vi "GetLocalClassPath.vi"(1 "full class name":string, 5 "error in (no error)":errorcluster) -> (15 "local class path":path, 16 "found?":bool, 19 "error out":errorcluster)   [LabVIEW 2017, in "G#RemoteProxy.lvclass"]
doc: "Returns the local class path on the computer."
uses:
  G#RemoteProxy.lvclass
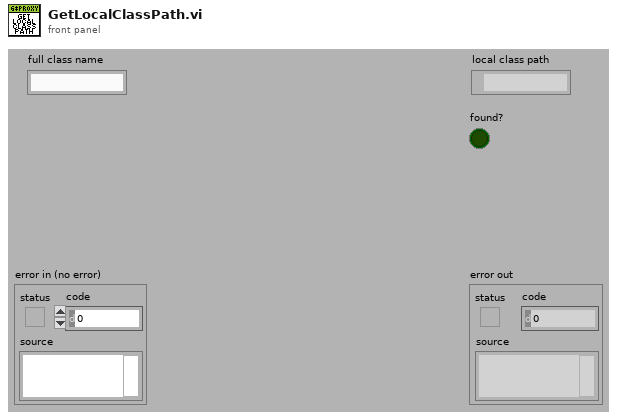
[diagram p1: front panel]
types:
  T1 = typedef "G#RemoteProxy.lvclass/ClassAttributesProxy.ctl" = cluster{"NoActiveProject":bool, "FullClassNames":string[], "FullClassPaths":path[], "RemoteRefs":refnum<class "G#Object.lvclass">[], "ProxyRefs":refnum<class "G#RemoteProxy.lvclass">[], "RemoteClassName":string[], "ProxyClassRefs":refnum<class "G#RemoteProxy.lvclass">[]}
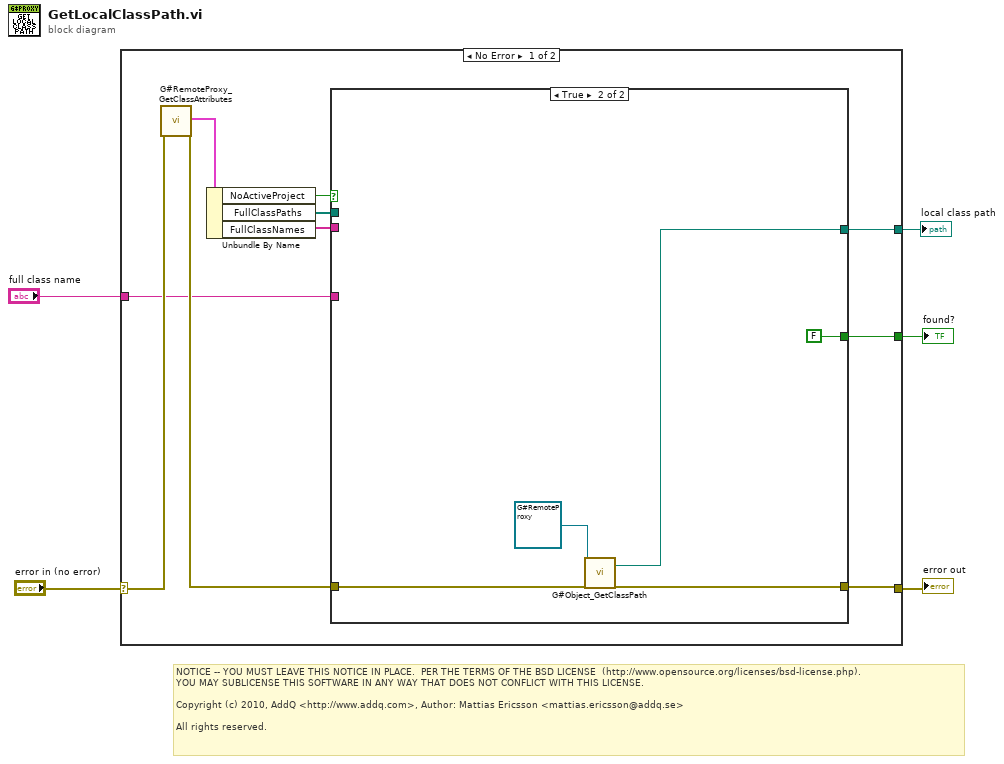
[diagram p0: block diagram]
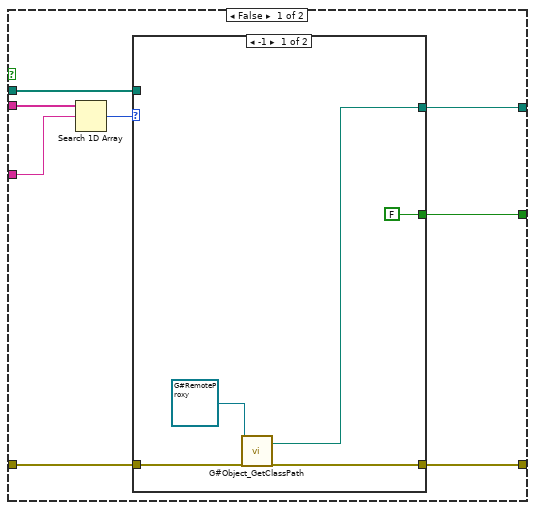
[diagram p2: hidden frame]
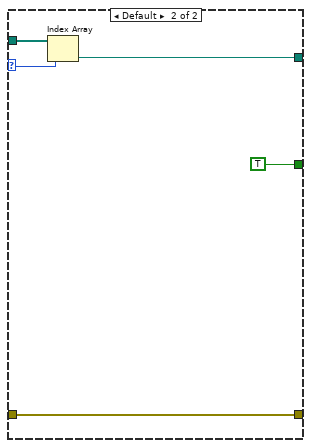
[diagram p3: hidden frame]
diagram:
  # "NOTICE -- YOU MUST LEAVE THIS NOTICE IN PLACE.  PER THE TERMS OF THE BSD LICENSE  (http://www.opensource.org/licenses/bsd-license.php).\nYOU MAY SUBLICENSE THIS SOFTWARE IN ANY WAY THAT DOES NOT CONFLICT WITH THIS LICENSE.\n\nCopyright (c) 2010, AddQ <http://www.addq.com>, Author: Mattias Ericsson <mattias.ericsson@addq.se>\n\nAll rights reserved."
  n1 = case shown="No Error" "error in (no error)" {
    selector: "error in (no error)" -> [w15 w39]
    tunnel: [w11 w39] -> w4
    tunnel: [w10 _] -> w3
    tunnel: "full class name" -> [w8 _]
    tunnel: [w6 _] -> w1
    frame No Error {
      n2 = call "G#RemoteProxy_GetClassAttributes.vi"("error in (no error)"=w15) -> ("class attributes"=w14:T1, "error out"=w12:errorcluster)  [unwired: 15 in, 2 out]
      n3 = Unbundle By Name(w14) -> ("NoActiveProject"=w13:bool, "FullClassPaths"=w7:path[], "FullClassNames"=w9:string[])
      n4 = case shown="True" w13 {
        tunnel: w12 -> [w17 w36]
        tunnel: [w16 w35] -> w11
        tunnel: [w18 FALSE] -> w10
        tunnel: w9 -> [w23 _]
        tunnel: w8 -> [w22 _]
        tunnel: w7 -> [w21 _]
        tunnel: [w19 w34] -> w6
        frame False {
          n5 = Search 1D Array(1D array=w23, element=w22) -> (index of element=w20:i32)  [unwired: 1 in]
          n6 = case shown="-1" w20 {
            selector: w20 -> [_ w32]
            tunnel: w21 -> [_ w33]
            tunnel: [w25 w31] -> w19
            tunnel: [FALSE TRUE] -> w18
            tunnel: w17 -> [w27 w29]
            tunnel: [w24 w29] -> w16
            frame -1 {
              n7 = call-dynamic "G#Object_GetClassPath.vi"("reference in"=refnum<class "G#RemoteProxy.lvclass"> refnum ("G#RemoteProxy.lvclass"), "error in (no error)"=w27) -> ("class path"=w25:path, "error out"=w24:errorcluster)  [unwired: 15 in, 1 out]
            }
            frame Default {
              n8 = Index Array(array=w33, index=w32) -> (element=w31:path)
            }
          }
        }
        frame True {
          n9 = call-dynamic "G#Object_GetClassPath.vi"("reference in"=refnum<class "G#RemoteProxy.lvclass"> refnum ("G#RemoteProxy.lvclass"), "error in (no error)"=w36) -> ("class path"=w34:path, "error out"=w35:errorcluster)  [unwired: 15 in, 1 out]
        }
      }
    }
    frame Error {
    }
  }
  "error out" <- w4
  "local class path" <- w1
  "found?" <- w3
